vi "_057.vi"() -> ()   [LabVIEW 2024]
panel:
  out "Waveform Graph":dbl[](graph)
  out "error out":errorcluster
  in  "Path":path
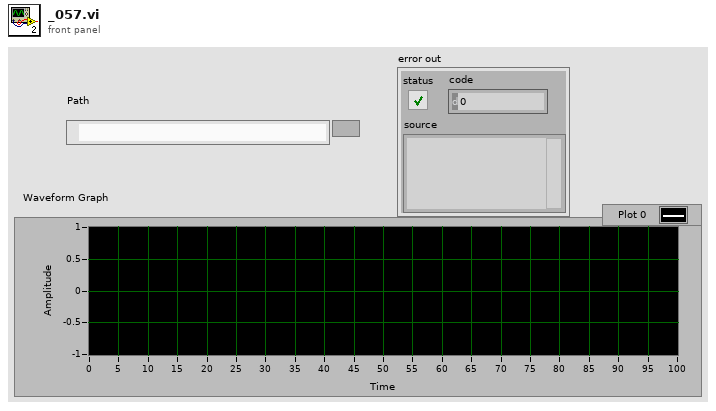
[diagram p1: front panel]
types:
  T1 = enum16{"open", "replace", "create", "open or create", "replace or create", "replace or create with confirmation"}
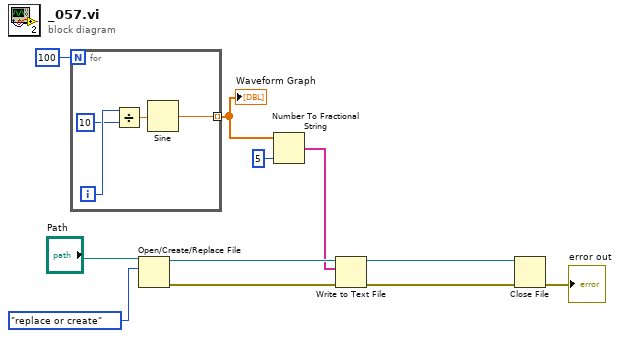
[diagram p0: block diagram]
diagram:
  n1 = for {
    N: 100 -> [_]
    tunnel: [w12] -> w3 mode=indexing
    i -> [w14]
    n2 = Divide(x=w14, y=10) -> (x/y=w15:dbl)
    n3 = Sine(x=w15) -> (sin(x)=w12:dbl)
  }
  "Waveform Graph" <- w3
  n4 = Open/Create/Replace File(file path (use dialog)="Path", operation (0:open)=T1."replace or create") -> (refnum out=w11:refnum<file>, error out=w9:errorcluster)  [unwired: 4 in, 1 out]
  n5 = Number To Fractional String(number=w3, precision (6)=i16 5) -> (F-format string=w2:string[])  [unwired: 2 in]
  n6 = Write to Text File(file (use dialog)=w11, text=w2, error in=w9) -> (refnum out=w10:refnum<file>, error out=w8:errorcluster)  [unwired: 1 in, 1 out]
  n7 = Close File(refnum=w10, error in=w8) -> (error out=→"error out":errorcluster)  [unwired: 1 out]
